vi "Move Elves - Unique Movement Order.vi"(0 "Elves in":T2(c390), 1 "Elves' Movement Proposals":map{T1, T1}(c390)) -> (2 "Elves out":T2(c390))   [LabVIEW 2020, in "AoC 2022.lvlib"]
uses:
  AoC 2022.lvlib
  Day 15 - Beacon Exclusion Zone/private/Location.ctl
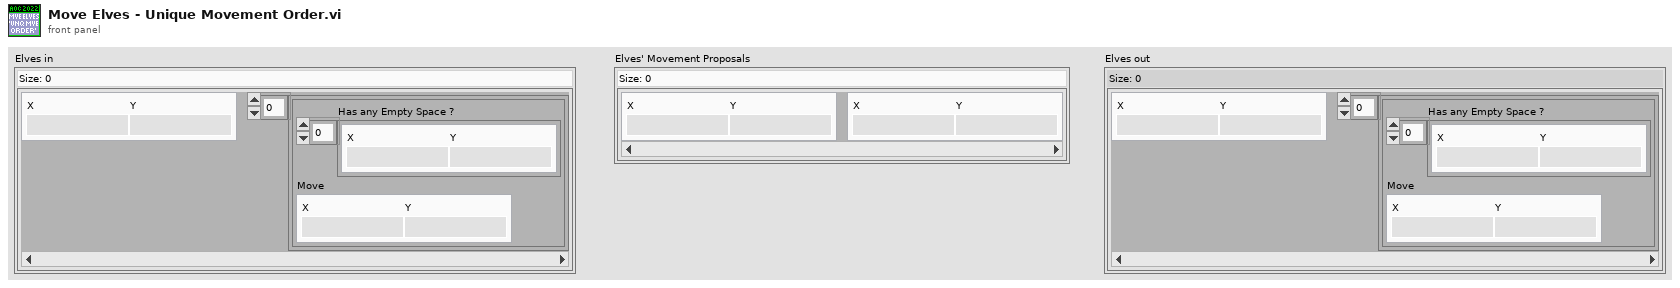
[diagram p1: front panel]
types:
  T1 = typedef "AoC 2022.lvlib/Location.ctl" = cluster{"X":i32, "Y":i32}
  T2 = map{T1, cluster{"Has any Empty Space ?":T1[], "Move":T1}[]}
  T3 = cluster{"Has any Empty Space ?":T1[], "Move":T1}[]
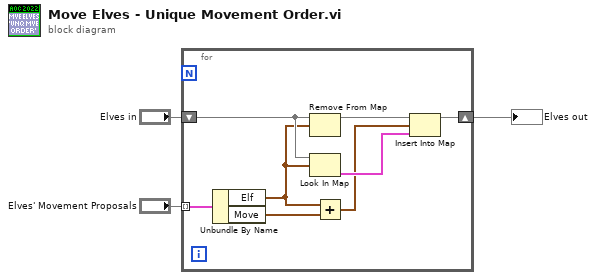
[diagram p0: block diagram]
diagram:
  n1 = for {
    tunnel: "Elves' Movement Proposals" -> [w11] mode=indexing
    shift-right: [w4] -> w1
    shift-left: "Elves in" -> [w7]
    n2 = Unbundle By Name(w11) -> ("Elf"=w6:T1, "Move"=w9:T1)
    n3 = Remove From Map(10:w6, 11:w7) -> (3:w5:T2)  [unwired: 2 out]
    n4 = Look In Map(map=w7, key=w6) -> (value=w10:T3)  [unwired: 1 in, 1 out]
    n5 = Add(x=w6, y=w9) -> (x+y=w8:T1)
    n6 = Insert Into Map(map in=w5, key=w8, value=w10) -> (map out=w4:T2)  [unwired: 2 out]
  }
  "Elves out" <- w1
